vi "Global camera setup trigger.vi"() -> ()   [LabVIEW 2020]
panel:
  out "Global camera setup trigger":bool
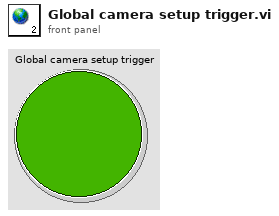
[diagram p1: front panel]
diagram:
